vi "DemoLED.vi"() -> ()   [LabVIEW 2009]
uses:
  <vilib>/NXT/Block Support/NXT_InputPort.ctl
  <vilib>/NXT/Dual Mode Library/Waits/Wait_Num(msec).vi
panel:
  in  "stop":bool
  # "Demo LED"
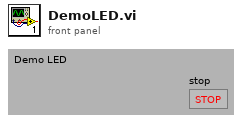
[diagram p1: front panel]
types:
  T1 = typedef "NXT_InputPort.ctl" = u8
  T2 = typedef "LVHSConnector.ctl" = cluster{"error":errorcluster, "address":string, "NXT #":i32, "Show Error":bool, "Connection":u16}
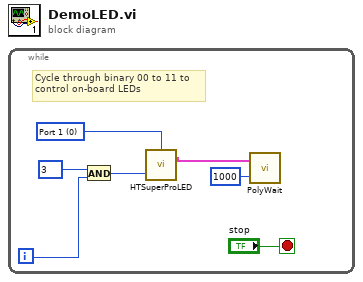
[diagram p0: block diagram]
diagram:
  n1 = while {
    i -> [w5]
    stop <- "stop" stop-if-true
    w2 = T1 0 items=["Port 1", "Port 2", "Port 3", "Port 4"] ("Port")
    # "Cycle through binary 00 to 11 to\ncontrol on-board LEDs"
    n2 = And(x=u8 3 ("Digital Control"), y=w5) -> (x .and. y?=w1:i32)
    n3 = call "HTSuperProLED.vi"("LED"=w1, "Port"=w2) -> ("NXT"=w3:T2)  [unwired: 3 in]
    n4 = call-poly <vilib>:"PolyWait.vi"("Time (100 msec)"=u32 1000, "NXT"=w3) -> ()  [unwired: 2 in, 1 out]
  }
